vi "Test Controller Fail to Verify User.vi"(8 "error in (no error)":errorcluster, 11 "Test Case In":refnum<class "Controller Test.lvclass">) -> (0 "error out":errorcluster, 3 "Test Case Out":refnum<class "Controller Test.lvclass">)   [LabVIEW 2020, in "Controller Test.lvclass"]
uses:
  Controller Test.lvclass
  C:/Program Files (x86)/National Instruments/LabVIEW 2020/vi.lib/Astemes/LUnit/Test Case.lvclass
  ATM Controller/State.ctl
  Account Database/Account Data.ctl
  <vilib>/Astemes/LUnit/Test Case.lvclass/Test Case.ctl
  01074fa8-ee8a-411d-bc8b-fc92c4f90959.vi
  <vilib>/Astemes/LUnit/Palette/Pass.vi
  <vilib>/Astemes/LUnit/Palette/Fail.vi
  <vilib>/Astemes/LUnit/Compare Variants.vi
  <vilib>/Astemes/LUnit/Describe Comparison.vi
  <vilib>/Astemes/LUnit/Set Assertion Type.vi
  <vilib>/Astemes/LUnit/Add test result.vi
  <vilib>/Astemes/LUnit/Variant to string.vi
  <vilib>/Astemes/LUnit/LUnit Record Assertion Result.vi
  <vilib>/Astemes/LUnit/LUnit Aggregate Assertion Results.vi
  <vilib>/Astemes/LUnit/Method Result/LUnit Merge Status.vi
  <vilib>/Astemes/LUnit/LUnit Concatenate result strings.vi
  <vilib>/Utility/Data Type/Get Type Information.vi
  <vilib>/Utility/LVClass/Get LV Class Name.vi
  ATM Controller/ATM Controller.lvclass
  Account Database/Account Database.lvclass
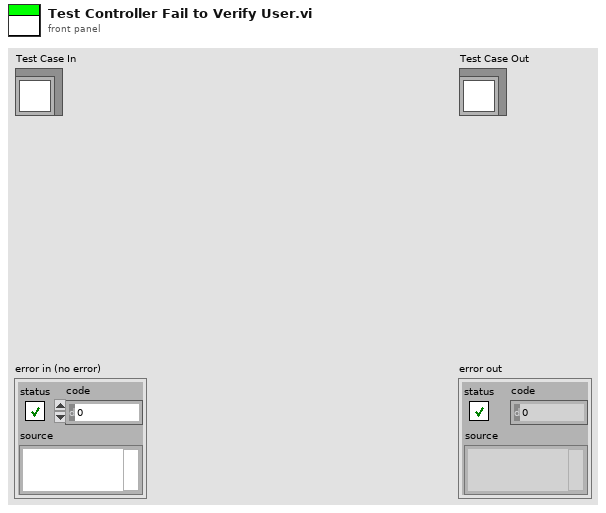
[diagram p1: front panel]
types:
  T1 = typedef "Account Database.lvclass/Account Data.ctl" = cluster{"Account Number":string, "First Name":string, "Last Name":string, "Account Balance":string}
  T2 = typedef "ATM Controller.lvclass/State.ctl" = enum16{"Start", "Card Inserted", "Verification Failed", "Verification Succeeded", "Depositing", "Terminate"}
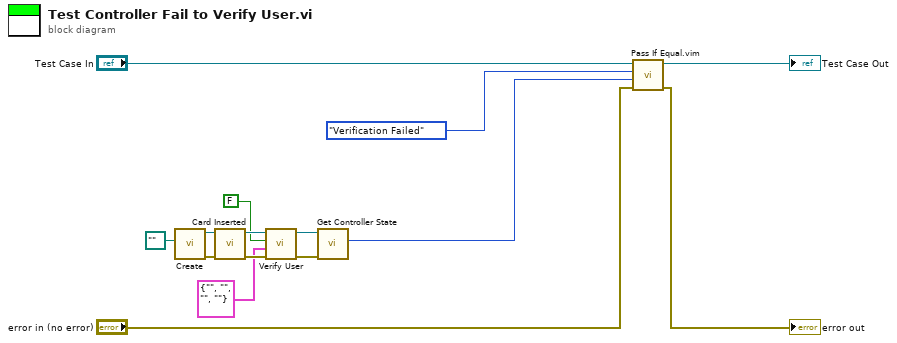
[diagram p0: block diagram]
diagram:
  n1 = call "Create.vi"("Data File"=path "") -> ("error out"=w11:errorcluster, "ATM Controller out"=w7:refnum<class "ATM Controller.lvclass">)  [unwired: 9 in]
  n2 = call "Card Inserted.vi"("error in (no error)"=w11, "ATM Controller in"=w7) -> ("error out"=w8:errorcluster, "ATM Controller out"=w5:refnum<class "ATM Controller.lvclass">)  [unwired: 8 in]
  n3 = call "Verify User.vi"("error in (no error)"=w8, "Account Data"=T1 {"Account Number"="", "First Name"="", "Last Name"="", "Account Balance"=""}, "Verified?"=FALSE, "ATM Controller in"=w5) -> ("error out"=w6:errorcluster, "ATM Controller out"=w4:refnum<class "ATM Controller.lvclass">)  [unwired: 6 in]
  n4 = call "Get Controller State.vi"("error in (no error)"=w6, "ATM Controller in"=w4) -> ("ATM State"=w10:T2)  [unwired: 7 in, 2 out]
  n5 = call "Pass If Equal.vim"("error in (no error)"="error in (no error)", "Actual"=w10, "Expected"=State."Verification Failed" ("ATM State"), "LUnit Test Case In"="Test Case In") -> ("error out"=→"error out":errorcluster, "LUnit Test Case Out"=→"Test Case Out":refnum<class "Controller Test.lvclass">)  [unwired: 6 in]
